vi "svx_SC Line Legend Visible.vi"(5 "selector.visible":bool, 8 "Tree":refnum<vi>, 9 "Shaft Centerline":refnum<vi>, 10 "Legend Width":u32, 11 "container":refnum<vi>) -> ()   [LabVIEW 2017, in "SVX SC Line.xctl"]
uses:
  <vilib>/addons/_XControls/Shaft Centerline/SVX SC Line.xctl
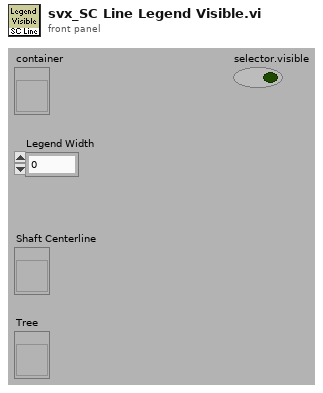
[diagram p1: front panel]
types:
  T1 = typedef "LVBoundsTypeDef.ctl" = cluster{"Width":u32, "Height":u32}
  T2 = typedef "LVRectTypeDef.ctl" = cluster{"Left":i16, "Top":i16, "Right":i16, "Bottom":i16}
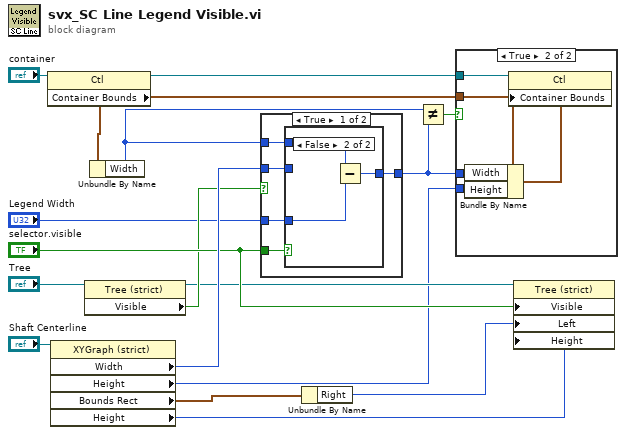
[diagram p0: block diagram]
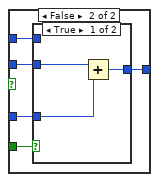
[diagram p4: hidden frame]
diagram:
  n1 = property class="Ctl"(reference="container") -> (reference out=w12:refnum<vi>, "Container Bounds"=w13:T1)  [unwired: 1 in, 1 out]
  n2 = property class="XYGraph (strict)"(reference="Shaft Centerline") -> ("Width"=w7:u32, "Height"=w1:u32, "Bounds Rect"=w9:T2, "Height"=w11:u32)  [unwired: 1 in, 2 out]
  n3 = property class="Tree (strict)"(reference="Tree") -> (reference out=w3:refnum<vi>, "Visible"=w4:bool)  [unwired: 1 in, 1 out]
  n4 = Unbundle By Name(w13) -> ("Width"=w8:u32)
  n5 = case shown="True" w4 {
    tunnel: "selector.visible" -> [w22 w31]
    tunnel: "Legend Width" -> [w21 w30]
    tunnel: [w20 w29] -> w17
    tunnel: w7 -> [w19 w28]
    tunnel: w8 -> [w18 w27]
    frame True {
      n6 = case shown="False" w22 {
        tunnel: w19 -> [_ _]
        tunnel: w21 -> [_ w26]
        tunnel: [w23 w25] -> w20
        tunnel: w18 -> [w23 w24]
        frame True {
        }
        frame False {
          n7 = Subtract(x=w24, y=w26) -> (x-y=w25:u32)
        }
      }
    }
    frame False {
      n8 = case shown="True" w31 {
        tunnel: w28 -> [w34 _]
        tunnel: w30 -> [w33 _]
        tunnel: [w32 w35] -> w29
        tunnel: w27 -> [_ w35]
        frame True {
          n9 = Add(x=w34, y=w33) -> (x+y=w32:u32)
        }
        frame False {
        }
      }
    }
  }
  n10 = Unbundle By Name(w9) -> ("Right"=w10:i16)
  n11 = Not Equal?(x=w8, y=w17) -> (x != y?=w16:bool)
  n12 = case shown="True" w16 {
    tunnel: w17 -> [_ w40]
    tunnel: w13 -> [_ w39]
    tunnel: w12 -> [_ w38]
    tunnel: w1 -> [_ w36]
    frame False {
    }
    frame True {
      n13 = Bundle By Name(cluster=w39, "Width"=w40, "Height"=w36) -> (w37:T1)
      n14 = property class="Ctl"(reference=w38, "Container Bounds"=w37) -> ()  [unwired: 1 in, 2 out]
    }
  }
  n15 = property class="Tree (strict)"(reference=w3, "Visible"="selector.visible", "Left"=w10, "Height"=w11) -> ()  [unwired: 1 in, 2 out]
